vi "testing2.vi"(11 "Numeric in":dbl) -> (3 "Numeric out":dbl)   [LabVIEW 2017]
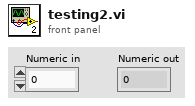
[diagram p1: front panel]
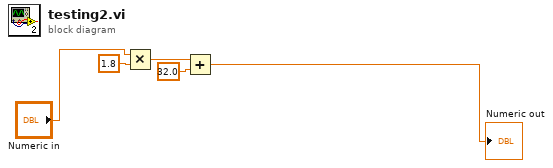
[diagram p0: block diagram]
diagram:
  n1 = Multiply(x="Numeric in", y=1.8 ("x*y")) -> (x*y=w3:dbl)
  n2 = Add(x=w3, y=32.0 ("x+y")) -> (x+y=→"Numeric out":dbl)
